vi "日志报警参数选择 (子VI).vi"(8 "error in (no error)":errorcluster caption="错误输入（无错误）", 11 "String输入":string) -> (0 "error out":errorcluster caption="错误输出", 3 "输出簇":T1)   [LabVIEW 2016]
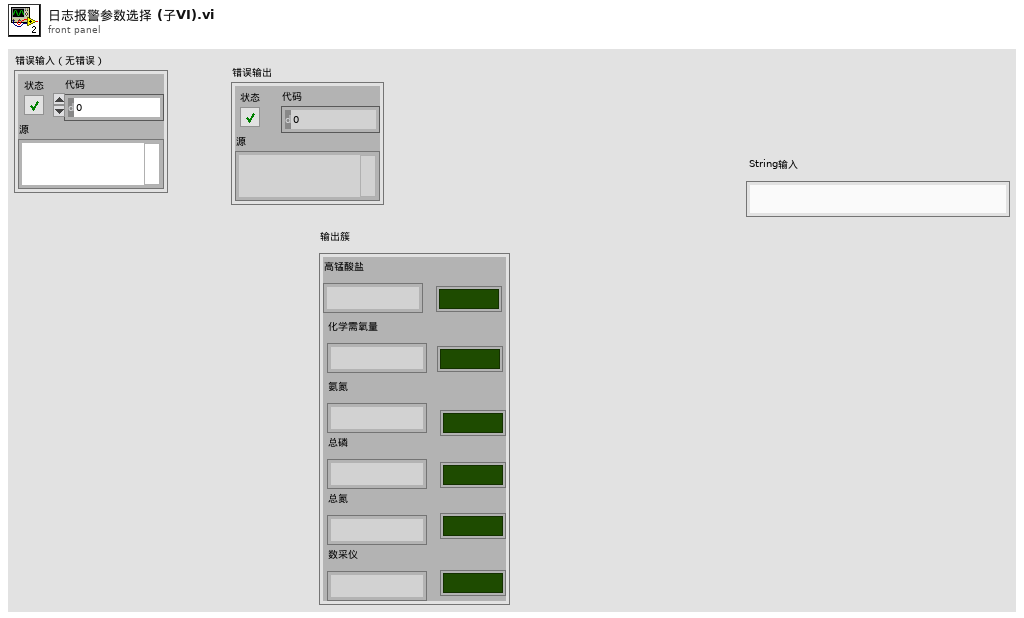
[diagram p1: front panel]
types:
  T1 = cluster{"高锰酸盐":string, "化学需氧量":string, "氨氮":string, "总磷":string, "总氮":string, "数采仪":string, "高锰酸盐":bool, "化学需氧量":bool, "氨氮":bool, "总磷":bool, "总氮":bool, "数采仪":bool}
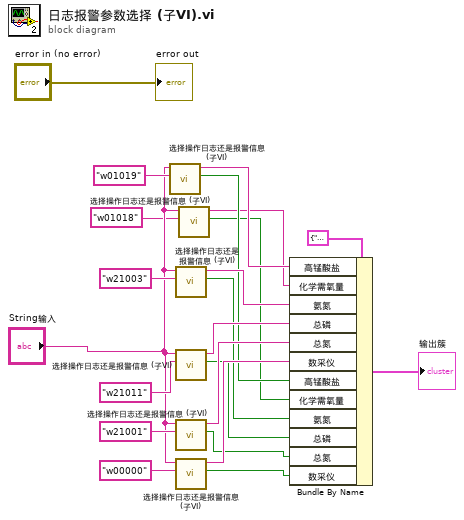
[diagram p0: block diagram]
diagram:
  n1 = call "选择操作日志还是报警信息 (子VI).vi"("搜索字符串"="w01019", "Value"="String输入") -> ("布尔"=w12:bool, "名称（未命名）"=w10:string)  [unwired: 8 in]
  n2 = call "选择操作日志还是报警信息 (子VI).vi"("搜索字符串"="w21003", "Value"="String输入") -> ("布尔"=w5:bool, "名称（未命名）"=w20:string)  [unwired: 8 in]
  n3 = call "选择操作日志还是报警信息 (子VI).vi"("搜索字符串"="w21011", "Value"="String输入") -> ("布尔"=w4:bool, "名称（未命名）"=w17:string)  [unwired: 8 in]
  n4 = call "选择操作日志还是报警信息 (子VI).vi"("搜索字符串"="w21001", "Value"="String输入") -> ("布尔"=w3:bool, "名称（未命名）"=w15:string)  [unwired: 8 in]
  n5 = call "选择操作日志还是报警信息 (子VI).vi"("搜索字符串"="w00000", "Value"="String输入") -> ("布尔"=w2:bool, "名称（未命名）"=w13:string)  [unwired: 8 in]
  n6 = call "选择操作日志还是报警信息 (子VI).vi"("搜索字符串"="w01018", "Value"="String输入") -> ("布尔"=w6:bool, "名称（未命名）"=w7:string)  [unwired: 8 in]
  n7 = Bundle By Name(cluster=T1 {"高锰酸盐"="", "化学需氧量"="", "氨氮"="", "总磷"="", "总氮"="", "数采仪"="", "高锰酸盐"=FALSE, "化学需氧量"=FALSE, "氨氮"=FALSE, "总磷"=FALSE, "总氮"=FALSE, "数采仪"=FALSE} ("输出簇"), "高锰酸盐"=w10, "化学需氧量"=w7, "氨氮"=w20, "总磷"=w17, "总氮"=w15, "数采仪"=w13, "高锰酸盐"=w12, "化学需氧量"=w6, "氨氮"=w5, "总磷"=w4, "总氮"=w3, "数采仪"=w2) -> (→"输出簇":T1)
  "error out" <- "error in (no error)"
